vi "Network_Map_(WIN).vi"(8 "Error In":errorcluster) -> (0 "Error Out":errorcluster, 3 "Terminal Output":string)   [LabVIEW 2017]
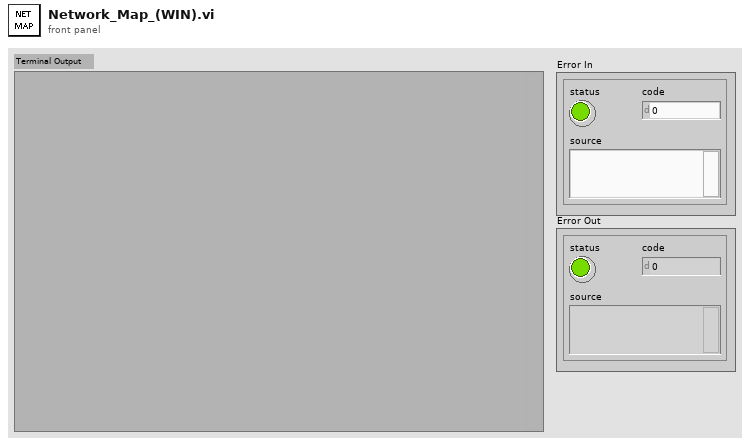
[diagram p1: front panel]
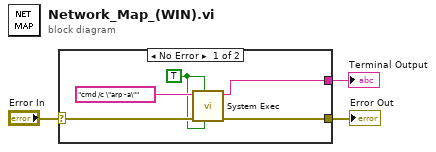
[diagram p0: block diagram]
diagram:
  n1 = case shown="No Error" "Error In" {
    selector: "Error In" -> [w7 w9]
    tunnel: [w6 w9] -> w2
    tunnel: [w5 _] -> w1
    frame No Error {
      w4 = TRUE ("wait until completion? (T)")
      n2 = call <vilib>:"System Exec.vi"("run minimized? (F)"=w4, "wait until completion? (T)"=w4, "error in (no error)"=w7, "command line"="cmd /c \"arp -a\"") -> ("error out"=w6:errorcluster, "standard output"=w5:string)  [unwired: 4 in, 2 out]
    }
    frame Error {
    }
  }
  "Error Out" <- w2
  "Terminal Output" <- w1
